vi "ready_pixelfly.vi"(3 "error in":errorcluster, 4 "Take Pictures":bool, 5 "PixelFly Controls":T1={"Acquitsition Settings"={"Buffer number"=1, "Size (Bytes)"=150, "initialized array"=array2048x1280[2621440 elements], "X Bin"=1, "Y Bin"=0, "Board Handle"=0, "Picture parameters"={"ccdxsize"=0, "ccdy"=0, "pictx"=0, "picty"=1, "bitspixel"=12}, "Buffer Out"=[]}, "Initialization"={"Exposure mode"=1, "exp time"=150, "exp level"=1, "gain"=0, "boardid in"=0, "offset"=0, "V bin"=0, "H bin"=0, "trigger"=TRUE, "Bit depth"=0}} {"Initialization"."Bit depth" items=["8", "12"]; "Initialization"."H bin" items=["1", "2"]; "Initialization"."V bin" items=["1", "2"]; "Initialization"."boardid in" min=0 max=3 step=1; "Initialization"."gain" items=["Low (X1)", "High (X2)"]; "Initialization"."exp level" min=0 max=255 step=1; "Initialization"."exp time" min=1 max=10000; "Initialization"."Exposure mode" items=["Asynch shutter", "Double shot", "Video mode", "Auto exposure"]}) -> (0 "error out":errorcluster)   [LabVIEW 2016]
doc: "Take a single PixelFly exposure and display the result as an intensity graph.This VI illustrates the basics of taking an exposure with the PixelFly camera. Use Ctrl-H to get help on any of the controls\n\nCopyright 2001, The Cooke Corporation."
uses:
  Controls/PixelFly/PixelFly_Control.ctl
  Controls/PixelFly/Acquisition Settings.ctl
  Controls/PixelFly/Bit_Depth_Enum.ctl
panel:
  out "Acquitsition Settings.Buffer number":i32
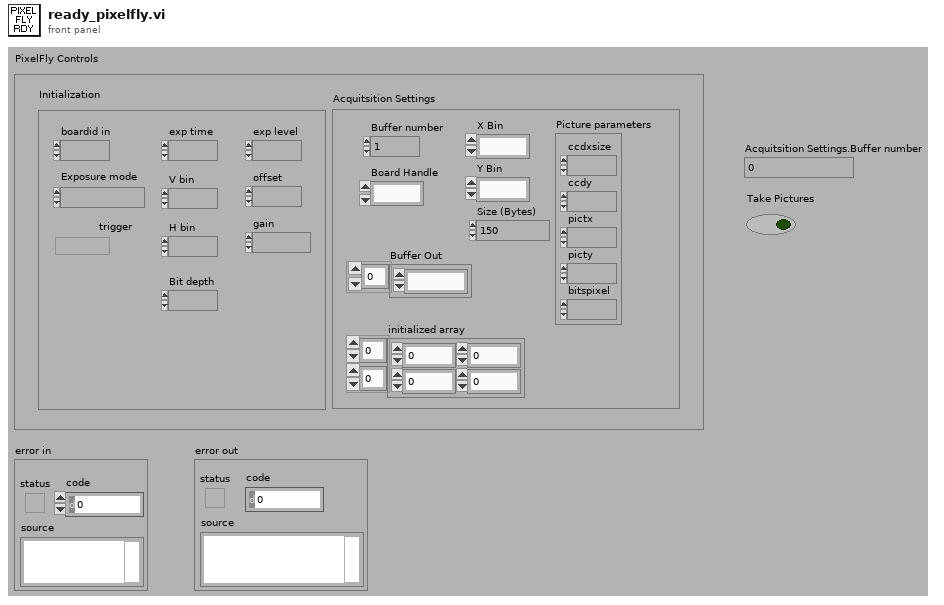
[diagram p1: front panel]
types:
  T1 = typedef "PixelFly_Control.ctl" = cluster{"Acquitsition Settings":T2, "Initialization":cluster{"Exposure mode":u16, "exp time":i32, "exp level":i32, "gain":i32, "boardid in":i32, "offset":i32, "V bin":i32, "H bin":i32, "trigger":bool, "Bit depth":T3}}
  T2 = typedef "Acquisition Settings.ctl" = cluster{"Buffer number":i32, "Size (Bytes)":i32, "initialized array":u16[][], "X Bin":i32, "Y Bin":i32, "Board Handle":u32, "Picture parameters":cluster{"ccdxsize":i32, "ccdy":i32, "pictx":i32, "picty":i32, "bitspixel":i32}, "Buffer Out":u16[]}
  T3 = typedef "Bit_Depth_Enum.ctl" = i32
  T4 = cluster{"Write":bool, "Write done":bool, "Queued":bool, "Cancelled":bool, "Select":bool, "Select done":bool, "Burst":bool, "Size":bool, "Event":bool, "Timeout":bool, "Open":i32, "Map":i32, "Exposure":i32[], "Offset":i32[], "Size":i32[], "Transfer":i32[], "Total Size":i32}
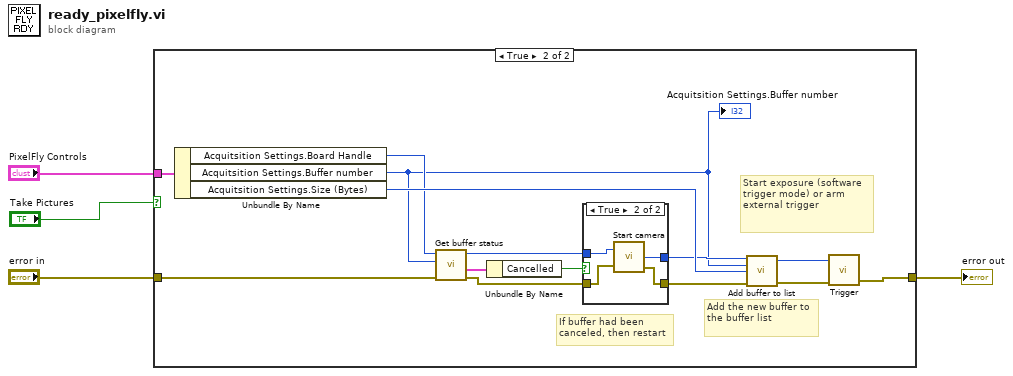
[diagram p0: block diagram]
diagram:
  n1 = case shown="True" "Take Pictures" {
    tunnel: "error in" -> [w5 w8]
    tunnel: [w5 w7] -> w3
    tunnel: "PixelFly Controls" -> [_ w6]
    frame False {
    }
    frame True {
      # "If buffer had been\ncanceled, then restart"
      # "Start exposure (software trigger mode) or arm external trigger"
      # "Add the new buffer to the buffer list"
      n2 = Unbundle By Name(w6) -> ("Acquitsition Settings.Board Handle"=w10:u32, "Acquitsition Settings.Buffer number"=w9:i32, "Acquitsition Settings.Size (Bytes)"=w18:i32)
      "Acquitsition Settings.Buffer number" <- w9
      n3 = call "Get buffer status.vi"("error in (no error)"=w8, "Buffer request"=w9, "Handle in"=w10) -> ("error out"=w11:errorcluster, "Buffer status"=w14:T4, "Handle out"=w12:u32)  [unwired: 1 in, 1 out]
      n4 = Unbundle By Name(w14) -> ("Cancelled"=w13:bool)
      n5 = case shown="True" w13 {
        tunnel: [w20 w25] -> w17
        tunnel: [w21 w24] -> w16
        tunnel: w12 -> [w21 w23]
        tunnel: w11 -> [w20 w22]
        frame False {
        }
        frame True {
          n6 = call "Start camera.vi"("Handle in"=w23, "error in (no error)"=w22) -> ("Handle out"=w24:u32, "error out"=w25:errorcluster)  [unwired: 1 out]
        }
      }
      n7 = call "Add buffer to list.vi"("Handle in"=w16, "Buffer in"=w9, "size"=w18, "error in (no error)"=w17) -> ("Handle out"=w15:u32, "error out"=w19:errorcluster)  [unwired: 9 in, 1 out]
      n8 = call "Trigger.vi"("Handle in"=w15, "error in (no error)"=w19) -> ("error out"=w7:errorcluster)  [unwired: 2 out]
    }
  }
  "error out" <- w3
